vi "Pre Launch Init.vi"(11 "Power Supply in":refnum<class "Power Supply.lvclass">) -> (0 "error out":errorcluster, 3 "Power Supply out":refnum<class "Power Supply.lvclass">)   [LabVIEW 2019, in "Power Supply.lvlib" / "Power Supply.lvclass"]
doc: "Initializes the panel actor. Creates the Panel Helper.\n\n----\nPlease see the following web address for additional documentation and tutorial information:\nhttp://www.mooregoodideas.com/mgi-panel-manager/\n\nAuthor: Derek Trepanier\n\nCopyright (c) 2018, Moore Good Ideas, Inc.\n\nAll rights reserved.\n\nRedistribution and use in source and binary forms, with or without modification, are permitted provided that the following conditions are met:\n\n * Redistributions of source code must retain the above copyright notice, this list of conditions and the following disclaimer.\n * Redistributions in binary form must reproduce the above copyright notice, this list of conditions and the following disclaimer in the documentation and/or other materials provided with the distribution.\n * Neither the name of Moore Good Ideas, Inc. nor the names of its contributors may be used to endorse or promote products derived from this software without specific prior written permission.\n\nTHIS SOFTWARE IS PROVIDED BY THE COPYRIGHT HOLDERS AND CONTRIBUTORS \"AS IS\" AND ANY EXPRESS OR IMPLIED WARRANTIES, INCLUDING, BUT NOT LIMITED TO, THE IMPLIED WARRANTIES OF MERCHANTABILITY AND FITNESS FOR A PARTICULAR PURPOSE ARE DISCLAIMED. IN NO EVENT SHALL THE COPYRIGHT OWNER OR CONTRIBUTORS BE LIABLE FOR ANY DIRECT, INDIRECT, INCIDENTAL, SPECIAL, EXEMPLARY, OR CONSEQUENTIAL DAMAGES (INCLUDING, BUT NOT LIMITED TO, PROCUREMENT OF SUBSTITUTE GOODS OR SERVICES; LOSS OF USE, DATA, OR PROFITS; OR BUSINESS INTERRUPTION) HOWEVER CAUSED AND ON ANY THEORY OF LIABILITY, WHETHER IN CONTRACT, STRICT LIABILITY, OR TORT (INCLUDING NEGLIGENCE OR OTHERWISE) ARISING IN ANY WAY OUT OF THE USE OF THIS SOFTWARE, EVEN IF ADVISED OF THE POSSIBILITY OF SUCH DAMAGE."
uses:
  Power Supply.lvclass
  Power Supply.lvclass/Power Supply.ctl
  Instrument/Instrument/Instrument.lvclass
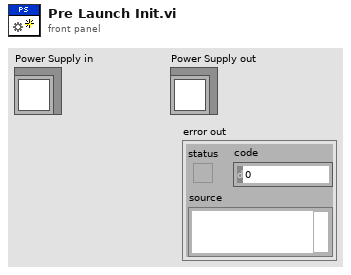
[diagram p1: front panel]
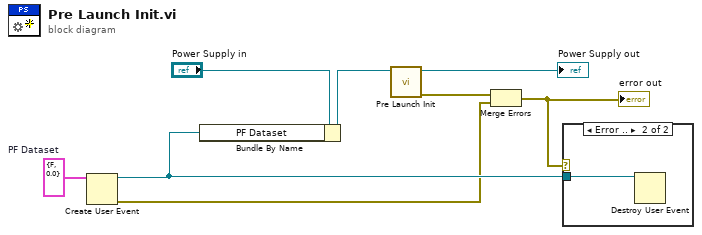
[diagram p0: block diagram]
diagram:
  w7 = cluster{"Run":bool, "Setpoint":dbl} {"Run"=FALSE, "Setpoint"=0.0}  # PF Dataset
  n1 = Create User Event(user event datatype=w7) -> (user event=w6:refnum<user-event>, error out=w4:errorcluster)  [unwired: 1 in]
  n2 = Bundle By Name(cluster="Power Supply in", "PF Dataset"=w6) -> (w2:refnum<class "Power Supply.lvclass">)
  n3 = call-parent "Pre Launch Init.vi"("Panel Actor in"=w2) -> ("error out"=w5:errorcluster, "Panel Actor out"=→"Power Supply out":refnum<class "Power Supply.lvclass">)  [unwired: 9 in]
  n4 = Merge Errors(w5, w4) -> (w1:errorcluster)
  "error out" <- w1
  n5 = case shown="Error .." w1 {
    tunnel: w6 -> [_ w9]
    frame No Error {
    }
    frame Error {
      n6 = Destroy User Event(user event=w9) -> ()  [unwired: 1 in, 1 out]
    }
  }
